vi "Read Check.vi"(8 "error in (no error)":errorcluster, 11 "Island Watch in":refnum<class "Island Watch.lvclass">) -> (0 "error out":errorcluster, 3 "Island Watch out":refnum<class "Island Watch.lvclass">)   [LabVIEW 2015, in "Island Watch Actor.lvlib" / "Island Watch.lvclass"]
uses:
  Island Watch.lvclass
  Island Watch.lvclass/Island Watch.ctl
  <vilib>/ActorFramework/Message Enqueuer/Message Priority.ctl
  <vilib>/ActorFramework/Actor/Actor.lvclass/Actor.ctl
  <vilib>/ActorFramework/Message Enqueuer/Message Enqueuer.lvclass/Message Enqueuer.ctl
  <vilib>/ActorFramework/Message Enqueuer/Init from Existing Queue.vi
  <vilib>/ActorFramework/Message Enqueuer/Enqueue.vi
  <vilib>/ActorFramework/Message Priority Queue/Priority Enqueue.vi
  <vilib>/ActorFramework/Message Enqueuer/Message Enqueuer.lvclass
  IED Actor/IED Messages/Engage Islanding Msg/Engage Islanding Msg.lvclass
  <vilib>/ActorFramework/Stop Msg/Stop Msg.lvclass
  <vilib>/Modbus/master/Modbus Master.lvclass
  <vilib>/ActorFramework/Actor/Actor.lvclass
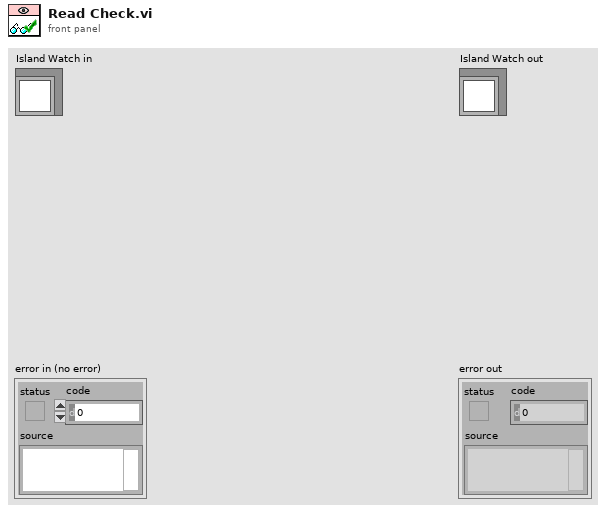
[diagram p1: front panel]
types:
  T1 = typedef "Actor Framework.lvlib/Message Enqueuer.lvclass/Message Priority.ctl" = enum16{"Low", "Normal", "High"}
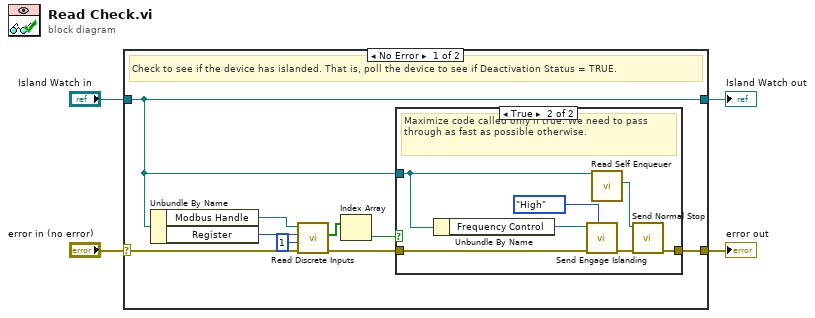
[diagram p0: block diagram]
diagram:
  n1 = case shown="No Error" "error in (no error)" {
    selector: "error in (no error)" -> [w8 w23]
    tunnel: [w7 w23] -> w3
    tunnel: [w5 w22] -> w1
    tunnel: "Island Watch in" -> [w5 w22]
    frame No Error {
      # "Check to see if the device has islanded. That is, poll the device to see if Deactivation Status = TRUE."
      n2 = Unbundle By Name(w5) -> ("Modbus Handle"=w9:refnum<class "Modbus Master.lvclass">, "Register"=w6:u16)
      n3 = call-dynamic "Read Discrete Inputs.vi"("error in (no error)"=w8, "number of discrete inputs"=u16 1 ("number of coils"), "starting address"=w6, "Modbus master in"=w9) -> ("error out"=w13:errorcluster, "discrete input values"=w11:bool[])  [unwired: 5 in, 1 out]
      n4 = Index Array(array=w11) -> (element=w12:bool)  [unwired: 1 in]
      n5 = case shown="True" w12 {
        tunnel: w13 -> [w14 w21]
        tunnel: [w14 w19] -> w7
        tunnel: w5 -> [_ w16]
        frame False {
          # "Do nothing."
        }
        frame True {
          # "Maximize code called only if true. We need to pass through as fast as possible otherwise."
          n6 = Unbundle By Name(w16) -> ("Frequency Control"=w17:refnum<class "Message Enqueuer.lvclass">)
          n7 = call "Send Engage Islanding.vi"("Message Priority (Normal)"=Message_Priority."High", "error in (no error)"=w21, "Message Enqueuer"=w17) -> ("error out"=w20:errorcluster)  [unwired: 7 in, 1 out]
          n8 = call <vilib>:"Read Self Enqueuer.vi"("Actor"=w16) -> ("Self Enqueuer"=w18:refnum<class "Message Enqueuer.lvclass">)  [unwired: 10 in]
          n9 = call <vilib>:"Send Normal Stop.vi"("error in (no error)"=w20, "Message Enqueuer"=w18) -> ("error out"=w19:errorcluster)  [unwired: 9 in]
        }
      }
    }
    frame Error {
    }
  }
  "error out" <- w3
  "Island Watch out" <- w1
